vi "DetermineFirstTrigger.vi"(9 "DAQ Channel Array":T8 {"Card Settings"."Start Time" format="%#_3p"; "Card Settings"."End Time" format="%#_3p"; "Card Settings"."Rate" format="%#_3p"}, 10 "RIOChannelArray":T1 {"Card Settings"."Digital High \nPass Filter k" items=["10"=21, "9"=19, "8"=17, "7"=15, "6"=13, "5"=11, "4"=9, "3"=7, "2"=5, "Off"=0]; "Card Settings"."Start Time" format="%#_3p"; "Card Settings"."End Time" format="%#_3p"; "Card Settings"."Rate" format="%#_3p"}, 11 "Timing Control Array":T13 {"Timing Sequence"."Pulse Width [s]" format="%#.2p"; "Timing Sequence"."Dt" format="%.2p"; "Timing Sequence"."Time" format="%.2p"}) -> (3 "first trigger":dbl)   [LabVIEW 2015]
uses:
  Controls/TimingControlArray.ctl
  Controls/TimingControl.ctl
  Controls/TimingControlChannel.ctl
  Controls/DAQ Channel Array.ctl
  Controls/DAQ Card-Channel Settings.ctl
  Controls/DAQ Card Channel Array.ctl
  Controls/DAQ Channel Settings.ctl
  Controls/DAQ Card Settings.ctl
  Controls/RIOCardArray.ctl
  Controls/RIOCardElement.ctl
  Controls/RIOCardChannelArray.ctl
  Controls/RIOChannelSettings.ctl
  Controls/RIOCardSettings.ctl
  <vilib>/userdefined/High Color/nirio_resource_hc.ctl
  Controls/DigitalHighPassFilter.ctl
panel:
  # "Channel                                                  Name                         Atten [dB]            Card Settings"
  # "Sampling Rate [1/s]"
  # "Start Time [s]"
  # "End Time [s]"
  # "Channel                                     Name                                                               Voltage Range                    Card Settings"
  # "Sampling Rate [1/s]"
  # "Start Time [s]"
  # "End Time [s]"
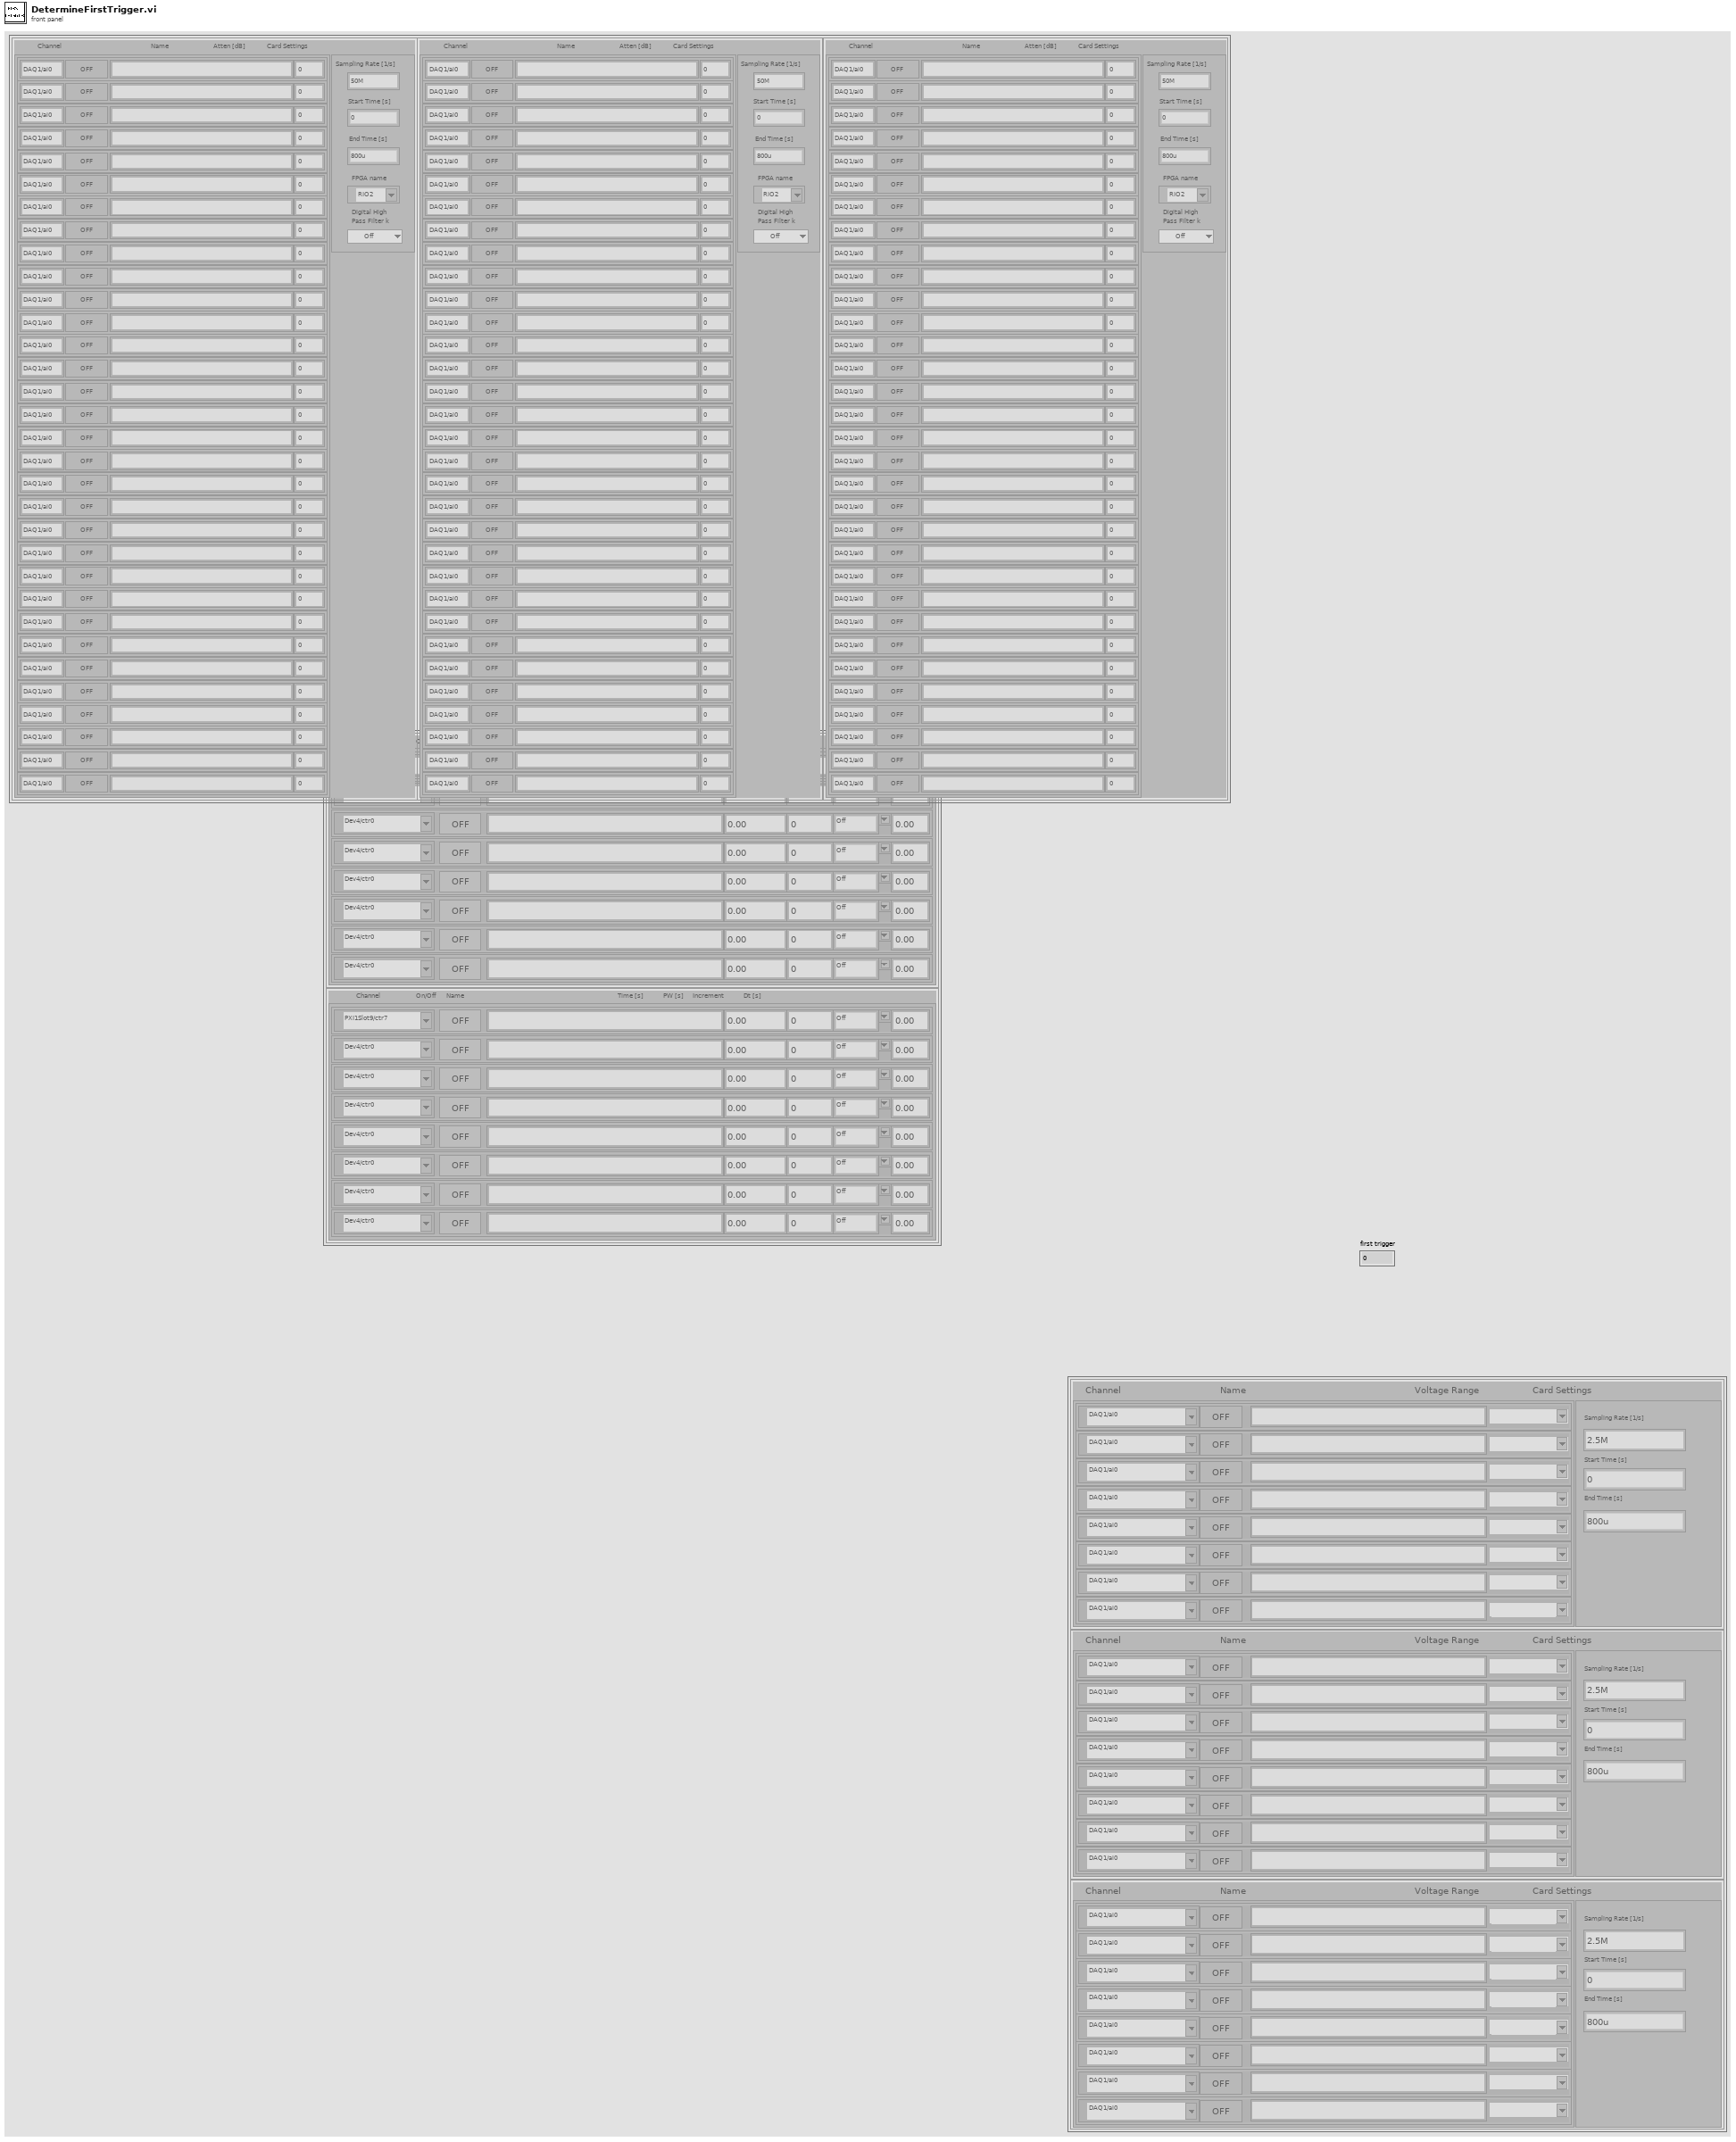
[diagram p1: front panel]
types:
  T1 = typedef "RIOCardArray.ctl" = T2[][]
  T2 = typedef "RIOCardElement.ctl" = cluster{"RIO Channel Array":T3, "Card Settings":T5}
  T3 = typedef "RIOCardChannelArray.ctl" = T4[]
  T4 = typedef "RIOChannelSettings.ctl" = cluster{"Active":bool, "Channel Name":string, "NI Name":string, "Attenutaion [dB]":i32}
  T5 = typedef "RIOCardSettings.ctl" = cluster{"Rate":dbl, "End Time":dbl, "Start Time":dbl, "FPGA name":T6, "Digital High \nPass Filter k":T7}
  T6 = typedef "nirio_resource_hc.ctl" = tag
  T7 = typedef "DigitalHighPassFilter.ctl" = u16
  T8 = typedef "DAQ Channel Array.ctl" = T9[]
  T9 = typedef "DAQ Card-Channel Settings.ctl" = cluster{"DAQ Channel Array":T10, "Card Settings":T12}
  T10 = typedef "DAQ Card Channel Array.ctl" = T11[]
  T11 = typedef "DAQ Channel Settings.ctl" = cluster{"Active":bool, "Channel Name":string, "Channel":tag, "Voltage Range":string}
  T12 = typedef "DAQ Card Settings.ctl" = cluster{"Rate":dbl, "End Time":dbl, "Start Time":dbl}
  T13 = typedef "TimingControlArray.ctl" = T14[]
  T14 = typedef "TimingControl.ctl" = cluster{"Timing Sequence":T15[]}
  T15 = typedef "TimingControlChannel.ctl" = cluster{"Active":bool, "counter":tag, "Channel Name":string, "Time":dbl, "Increment":string, "Dt":dbl, "Pulse Width [s]":dbl}
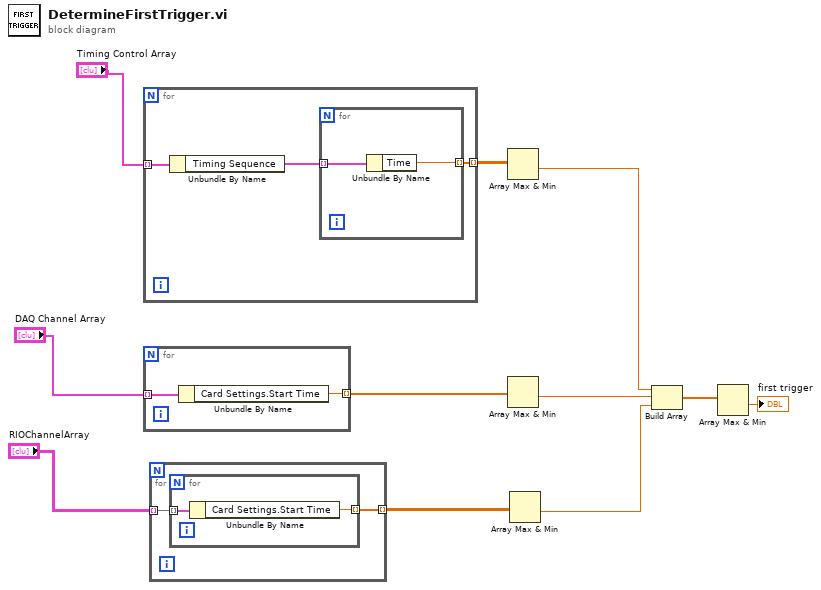
[diagram p0: block diagram]
diagram:
  n1 = for {
    tunnel: "Timing Control Array" -> [w14] mode=indexing
    tunnel: [w12] -> w10 mode=indexing
    n2 = Unbundle By Name(w14) -> ("Timing Sequence"=w13:T15[])
    n3 = for {
      tunnel: w13 -> [w16] mode=indexing
      tunnel: [w15] -> w12 mode=indexing
      n4 = Unbundle By Name(w16) -> ("Time"=w15:dbl)
    }
  }
  n5 = for {
    tunnel: "DAQ Channel Array" -> [w18] mode=indexing
    tunnel: [w17] -> w7 mode=indexing
    n6 = Unbundle By Name(w18) -> ("Card Settings.Start Time"=w17:dbl)
  }
  n7 = for {
    tunnel: "RIOChannelArray" -> [w19] mode=indexing
    tunnel: [w20] -> w6 mode=indexing
    n8 = for {
      tunnel: [w22] -> w20 mode=indexing
      tunnel: w19 -> [w21] mode=indexing
      n9 = Unbundle By Name(w21) -> ("Card Settings.Start Time"=w22:dbl)
    }
  }
  n10 = Array Max & Min(array=w10) -> (min value=w5:dbl)  [unwired: 3 out]
  n11 = Array Max & Min(array=w7) -> (min value=w4:dbl)  [unwired: 3 out]
  n12 = Array Max & Min(array=w6) -> (min value=w3:dbl)  [unwired: 3 out]
  n13 = Build Array(w5, w4, w3) -> (w2:dbl[])
  n14 = Array Max & Min(array=w2) -> (min value=→"first trigger":dbl)  [unwired: 3 out]
